vi "InfoResult.vi"(8 "error in":errorcluster, 11 "Result Step":T1) -> (0 "error out":errorcluster, 3 "Info Test":string)   [LabVIEW 2019]
doc: "Formatta le informazioni principali del risultato dell'update in una info box più leggibile"
uses:
  ByteQXAPIBase/TypeDef/UpdateLimsTestStepData.ctl
  ByteQXAPIBase/ByteQXAPIBase.lvclass
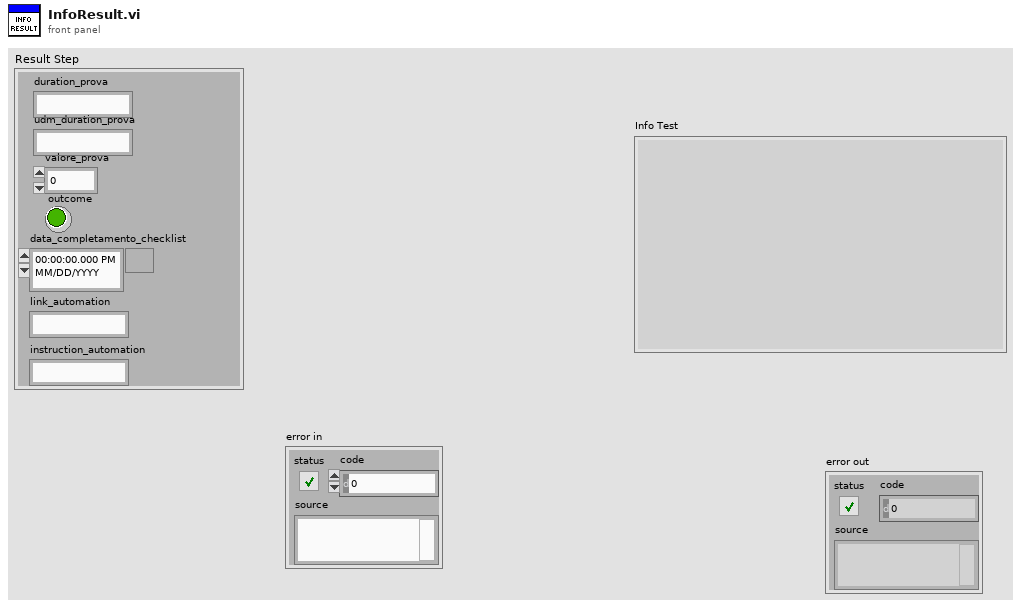
[diagram p1: front panel]
types:
  T1 = typedef "ByteQXWebAPI.lvlib/ByteQXAPIBase.lvclass/UpdateLimsTestStepData.ctl" = cluster{"outcome":bool, "data_completamento_checklist":timestamp, "udm_duration_prova":string, "valore_prova":dbl, "link_automation":string, "instruction_automation":string, "duration_prova":string}
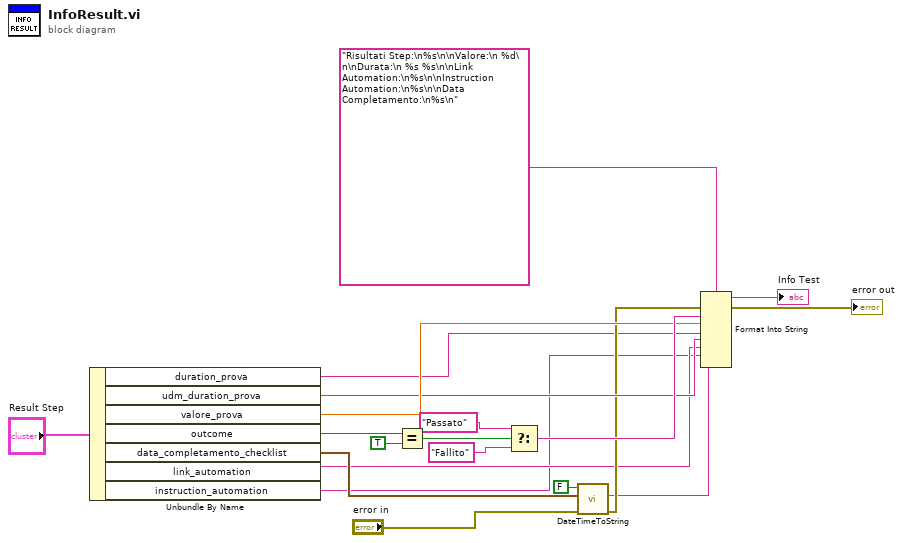
[diagram p0: block diagram]
diagram:
  n1 = Unbundle By Name("Result Step") -> ("duration_prova"=w6:string, "udm_duration_prova"=w11:string, "valore_prova"=w12:dbl, "outcome"=w20:bool, "data_completamento_checklist"=w16:timestamp, "link_automation"=w5:string, "instruction_automation"=w4:string)
  n2 = Equal?(x=w20, y=TRUE) -> (x = y?=w19:bool)
  n3 = Select(t="Passato" ("y"), s=w19, f="Fallito" ("y")) -> (s? t:f=w13:string)
  n4 = call "DateTimeToString.vi"("error in"="error in", "current time"=w16, "include Time?"=FALSE ("Time")) -> ("error out"=w10:errorcluster, "date string"=w3:string)  [unwired: 7 in]
  n5 = Format Into String(format string="Risultati Step:\n%s\n\nValore:\n %d\n\nDurata:\n %s %s\n\nLink Automation:\n%s\n\nInstruction Automation:\n%s\n\nData Completamento:\n%s\n", error in=w10, w13, w12, w6, w11, w5, w4, w3) -> (resulting string=→"Info Test":string, error out=→"error out":errorcluster)  [unwired: 1 in]
